vi "Snap Data.vi"(8 "error in":errorcluster, 11 "5105 in":refnum<class "5105.lvclass">) -> (0 "error out":errorcluster, 1 "wfm":waveform(dbl)[](array[waveform]), 2 "Auto Trigger":bool, 3 "5105 out":refnum<class "5105.lvclass">, 5 "Timeout":bool)   [LabVIEW 2019, in "5105.lvlib" / "5105.lvclass"]
uses:
  5105.lvclass
  C:/Users/Public/Documents/Development/builds/Instruments/Oscilloscope.lvlibp/Oscilloscope.lvclass
  C:/Users/Public/Documents/Development/builds/Engine/Monitored Actor.lvlibp/Monitored Actor/Monitored Actor/Monitored Actor.lvclass
  builds/Instruments/Oscilloscope.lvlibp/Accessors/Read Channel Setting.vi
  Accessors/Read Local Resource.vi
  builds/Engine/Monitored Actor.lvlibp/Monitored Actor/Monitored Actor/Read Actor Label.vi
  <instrlib>/niScope/Acquire/Fetch/niScope Multi Fetch WDT.vi
  Accessors/Write Local Resource.vi
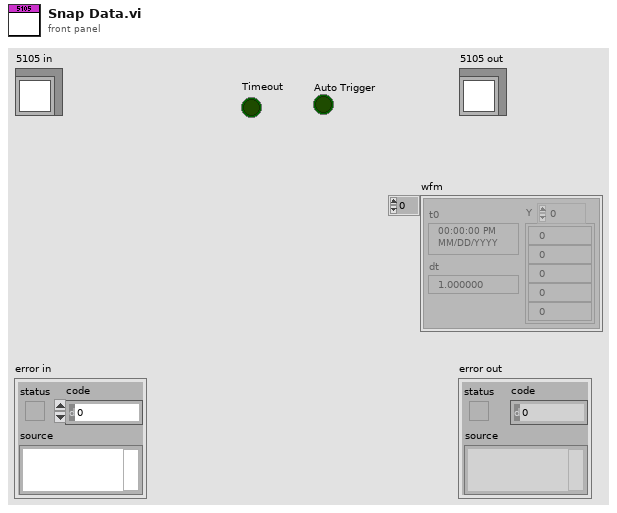
[diagram p1: front panel]
types:
  T1 = typedef "Oscilloscope.lvlibp/Oscilloscope.lvclass/Channel Settings.ctl" = cluster{"Amplitude":dbl, "Vertical Coupling":T2, "Probe Attenuation":dbl, "Enable?":bool, "Maximum Input Frequency":dbl, "Input Impedance":u16, "Timeout (s)":dbl}
  T2 = typedef "Oscilloscope.lvlibp/Oscilloscope.lvclass/Vertical Coupling.ctl" = enum16{"AC", "DC", "Ground"}
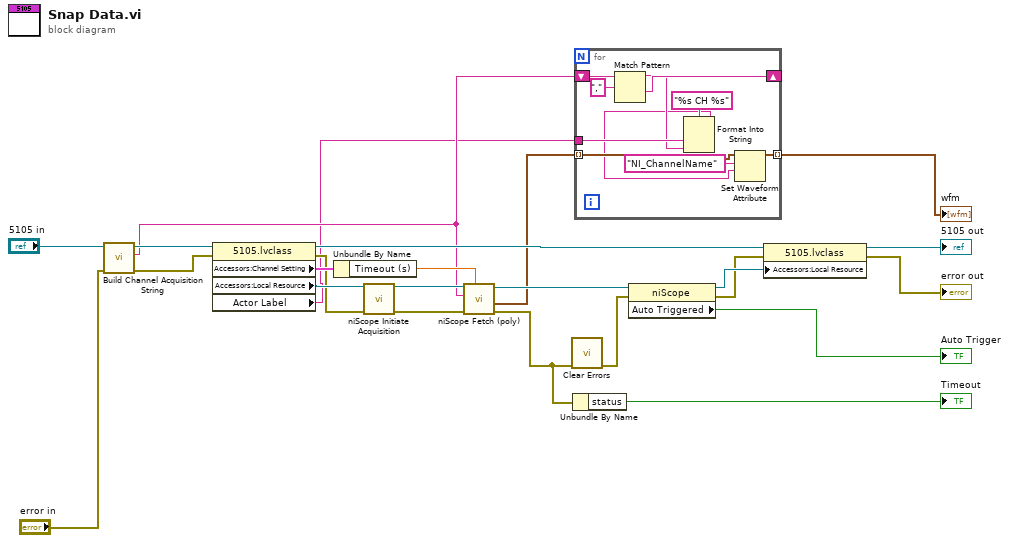
[diagram p0: block diagram]
diagram:
  n1 = call "Build Channel Acquisition String.vi"("error in (no error)"="error in", "5105 in"="5105 in") -> ("error out"=w20:errorcluster, "Channel Acquisition String"=w3:string, "5105 out"=w21:refnum<class "5105.lvclass">)  [unwired: 7 in]
  n2 = property class="5105.lvclass"(reference=w21, error in=w20) -> (reference out=w12:refnum<class "5105.lvclass">, error out=w18:errorcluster, "Accessors:Channel Setting"=w23:T1, "Accessors:Local Resource"=w24:refnum<k15>, "Actor Label"=w2:string)
  n3 = Unbundle By Name(w23) -> ("Timeout (s)"=w6:dbl)
  n4 = call <instrlib>:"niScope Initiate Acquisition.vi"("instrument handle"=w24, "error in"=w18) -> ("instrument handle out"=w8:refnum<k15>, "error out"=w9:errorcluster)  [unwired: 12 in]
  n5 = call-poly <instrlib>:"niScope Fetch (poly).vi"("timeout"=w6, "error in"=w9, "channels"=w3, "instrument handle"=w8) -> ("error out"=w5:errorcluster, "wfm"=w4:waveform(dbl)[], "instrument handle out"=w7:refnum<k15>)  [unwired: 4 in, 1 out]
  n6 = call <vilib>:"Clear Errors.vi"("error in (no error)"=w5) -> ("error out"=w17:errorcluster)  [unwired: 5 in, 1 out]
  n7 = Unbundle By Name(w5) -> ("status"=→"Timeout":bool)
  n8 = for {
    tunnel: w4 -> [w30] mode=indexing
    shift-right: [w33] -> _
    shift-left: w3 -> [w34]
    tunnel: w2 -> [w32]
    tunnel: [w29] -> w1 mode=indexing
    n9 = Match Pattern(string=w34, regular expression=",") -> (before substring=w31:string, after substring=w33:string)  [unwired: 1 in, 2 out]
    n10 = Format Into String(format string="%s CH %s", w32, w31) -> (resulting string=w25:string)  [unwired: 2 in, 1 out]
    n11 = Set Waveform Attribute(5:w25, 6:"NI_ChannelName" ("name"), 7:w30) -> (3:w29:waveform(dbl))  [unwired: 1 in, 2 out]
  }
  "wfm" <- w1
  n12 = property on="Property Node" class="niScope"(reference=w7, error in=w17) -> (reference out=w14:refnum<k15>, error out=w13:errorcluster, "Auto Triggered"=→"Auto Trigger":bool)
  n13 = property class="5105.lvclass"(reference=w12, error in=w13, "Accessors:Local Resource"=w14) -> (reference out=→"5105 out":refnum<class "5105.lvclass">, error out=→"error out":errorcluster)
